vi "Test Count Errors on Broken.vi"(8 "error in (no error)":errorcluster, 11 "Result Model Tests in":refnum<class "Result Model Statistics.lvclass">) -> (0 "error out":errorcluster, 3 "Result Model Tests out":refnum<class "Result Model Statistics.lvclass">)   [LabVIEW 2020, in "Result Model Statistics.lvclass"]
uses:
  Result Model Statistics.lvclass
  206db1ee-aa99-40b9-8881-171f2a77c34b.vi
  source/User Interface/Result Model/Result Model.lvclass
  source/Core/Result/Type.ctl
  source/Core/Result/Result.lvlib
  source/Core/Result/Status.ctl
  source/Core/Result/Result.ctl
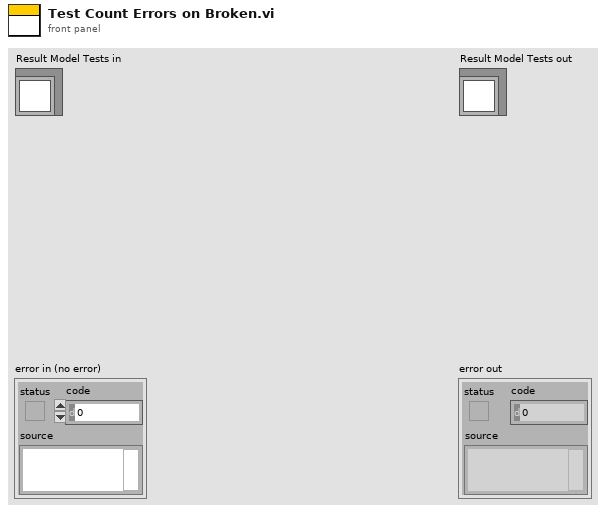
[diagram p1: front panel]
types:
  T1 = typedef "Result.lvlib/Result.ctl" = cluster{"Name":string, "Description":string, "Status":T2, "Result Type":T3, "Execution Time":dbl, "Data":cluster{"Expected":variant, "Actual":variant, "Delta":variant}}
  T2 = typedef "Result.lvlib/Status.ctl" = enum16{"", "Passed", "Failed", "Error", "Skipped", "Setup Error", "Broken", "Teardown Error"}
  T3 = typedef "Result.lvlib/Type.ctl" = enum16{"Test Case", "Test Suite", "Test Run", "Pass", "Fail", "Skip", "Pass if", "Fail if", "Pass if Error", "Fail if Error", "Pass if Equal", "Fail if Equal"}
  T4 = typedef "Result Model.lvclass/Statistics.ctl" = cluster{"Method Count":u32, "Executed Methods":u32, "Passed Methods":u32, "Failed Methods":u32, "Method Errors":u32, "Skipped Method":u32, "Progress [%]":dbl}
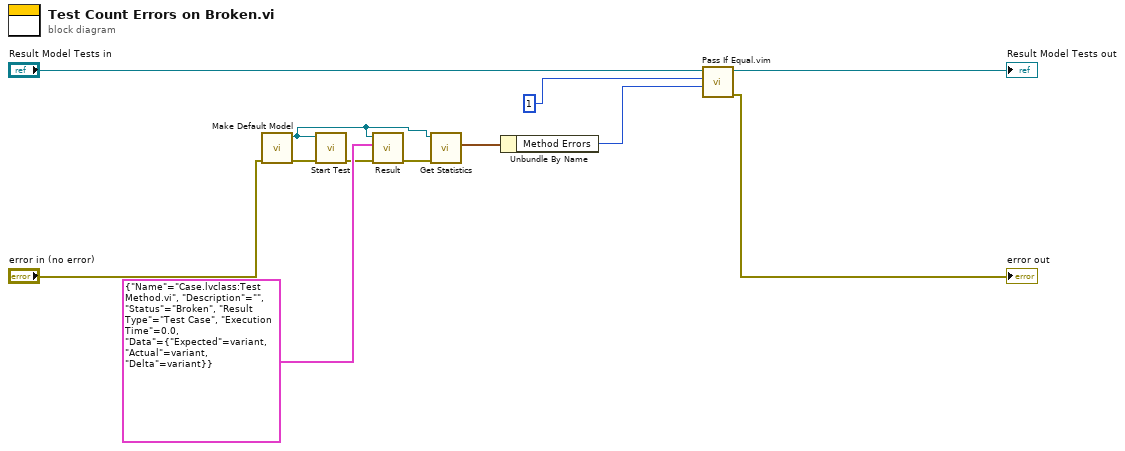
[diagram p0: block diagram]
diagram:
  n1 = call "Make Default Model.vi"("error in (no error)"="error in (no error)") -> ("error out"=w4:errorcluster, "Result Model out"=w1:refnum<class "Result Model.lvclass">)  [unwired: 9 in]
  n2 = call "Start Test.vi"("error in (no error)"=w4, "Result Model by Reference In"=w1) -> ("error out"=w3:errorcluster)  [unwired: 9 in]
  n3 = call-dynamic "Result.vi"("error in (no error)"=w3, "Results"=T1 {"Name"="Case.lvclass:Test Method.vi", "Description"="", "Status"=enum."Broken", "Result Type"=enum."Test Case", "Execution Time"=0.0, "Data"={"Expected"=variant, "Actual"=variant, "Delta"=variant}} ("Result"), "Result Model by Reference In"=w1) -> ("error out"=w2:errorcluster)  [unwired: 8 in]
  n4 = call "Get Statistics.vi"("error in (no error)"=w2, "Result Model in"=w1) -> ("Results"=w8:T4)  [unwired: 8 in, 1 out]
  n5 = Unbundle By Name(w8) -> ("Method Errors"=w7:u32)
  n6 = call "Pass If Equal.vim"("Actual"=w7, "Expected"=u32 1 ("Method Count"), "LUnit Test Case In"="Result Model Tests in") -> ("error out"=→"error out":errorcluster, "LUnit Test Case Out"=→"Result Model Tests out":refnum<class "Result Model Statistics.lvclass">)  [unwired: 7 in]
